vi "Broadcast Order State.vi"(8 "error in (no error)":errorcluster, 11 "Customer in":refnum<class "Customer.lvclass">) -> (0 "error out":errorcluster, 3 "Customer out":refnum<class "Customer.lvclass">)   [LabVIEW 2020, in "Customer.lvclass"]
uses:
  Customer.lvclass
  Customer.lvclass/Customer.ctl
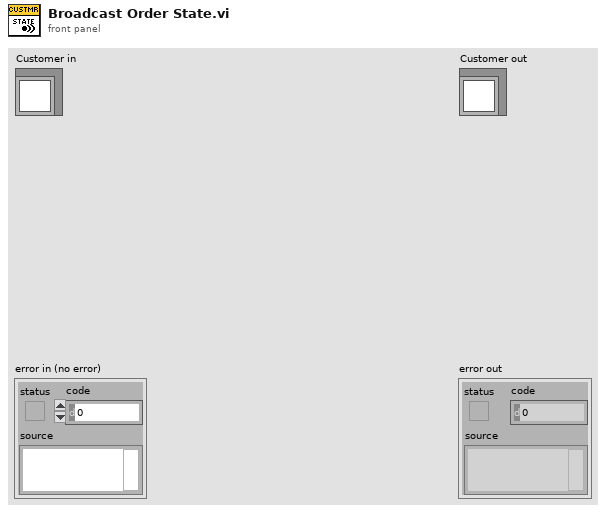
[diagram p1: front panel]
types:
  T1 = typedef "Customer.lvclass/Order State.ctl" = cluster{"Order In Progress?":bool, "Order Number":u32, "Order Price":dbl, "Items Ordered":u32, "Items Received":u32, "Items Picked Up":string}
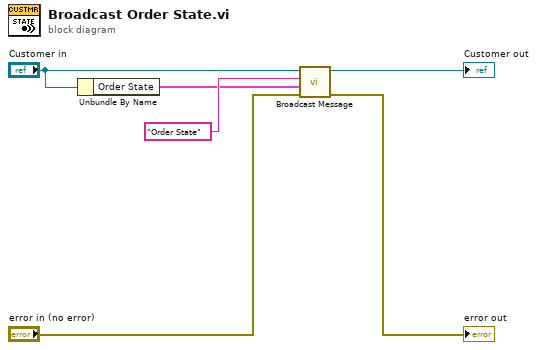
[diagram p0: block diagram]
diagram:
  n1 = Unbundle By Name("Customer in") -> ("Order State"=w1:T1)
  n2 = call-dynamic "Broadcast Message.vi"("error in (no error)"="error in (no error)", "Message Data"=w1, "Message"="Order State", "Rig Process In"="Customer in") -> ("error out"=→"error out":errorcluster, "Rig Process Out"=→"Customer out":refnum<class "Customer.lvclass">)  [unwired: 6 in]
